vi "Inverse_Kinematics_to_Counts.vi"(3 "pz":dbl, 4 "py":dbl, 5 "px":dbl) -> (0 "j3":i32, 1 "j2":i32, 2 "j1":i32)   [LabVIEW 2010]
doc: "This VI converts the desired tool tip position (px,py,pz) [mm] into joint motions of theta 1, theta 2, and theta 3 [counts]."
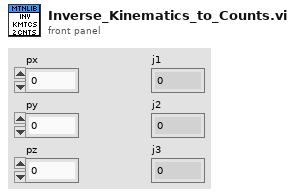
[diagram p1: front panel]
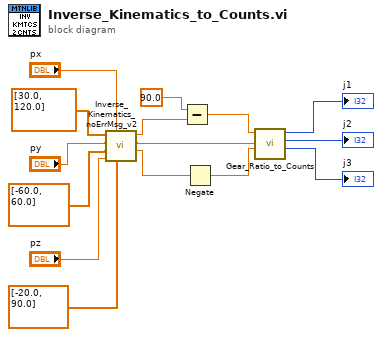
[diagram p0: block diagram]
diagram:
  n1 = call "Inverse_Kinematics_noErrMsg_v2.vi"("B3"=dbl[] [-20.0, 90.0], "px"="px", "pz"="pz", "B2"=dbl[] [-60.0, 60.0], "py"="py", "B1"=dbl[] [30.0, 120.0]) -> ("theta 3"=w3:dbl, "theta 2"=w2:dbl, "theta 1"=w1:dbl)  [unwired: 1 in]
  n2 = Subtract(x=90.0, y=w1) -> (x-y=w14:dbl)
  n3 = Negate(x=w3) -> (-x=w13:dbl)
  n4 = call "Gear_Ratio_to_Counts.vi"("theta 3"=w13, "theta 2"=w2, "theta 1"=w14) -> ("j3"=→"j3":i32, "j2"=→"j2":i32, "j1"=→"j1":i32)  [unwired: 1 in, 1 out]
